vi "Intake In Angle.vi"(8 "Tolerance":dbl, 9 "Target":dbl, 10 "Actual":dbl) -> (1 "In Range?":bool)   [LabVIEW 2016]
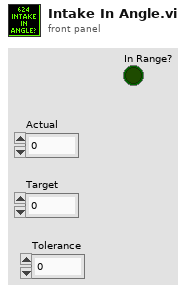
[diagram p1: front panel]
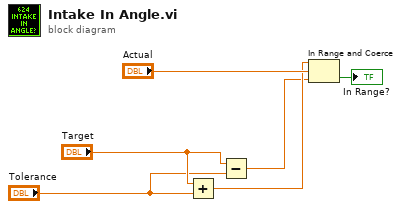
[diagram p0: block diagram]
diagram:
  n1 = Add(x="Target", y="Tolerance") -> (x+y=w5:dbl)
  n2 = Subtract(x="Target", y="Tolerance") -> (x-y=w2:dbl)
  n3 = In Range and Coerce(upper limit=w5, x="Actual", lower limit=w2) -> (In Range?=→"In Range?":bool)  [unwired: 1 out]
